vi "stdin.vi"() -> (0 "error out":errorcluster, 1 "bytes read":i32, 2 "eof?":bool, 3 "data":string)   [LabVIEW 2014]
doc: "Reads a number of bytes from stdin. Returns the results in the data string output. The VI does not wait for data, so if the amount of data is not available, the VI returns any available data."
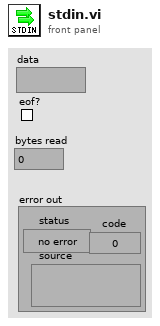
[diagram p1: front panel]
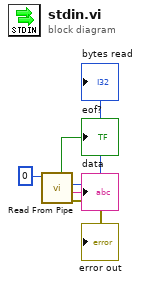
[diagram p0: block diagram]
diagram:
  n1 = call <vilib>:"Read From Pipe.vi"("file descriptor"=0) -> ("eof?"=→"eof?":bool, "bytes read"=→"bytes read":i32, "data"=→"data":string, "error out"=→"error out":errorcluster)  [unwired: 3 in, 1 out]
